vi "Event Handle Loop_Close Button.vi"(8 "error in (no error)":errorcluster, 10 "Label":string[](array[string]), 11 "QMenu Class in":refnum<class "QMenu Class.lvclass">) -> (0 "error out":errorcluster, 3 "QMenu Class out":refnum<class "QMenu Class.lvclass">)   [LabVIEW 2020, in "QTab.lvlib" / "QMenu Class.lvclass"]
uses:
  QMenu Class.lvclass
  QMenu Class.lvclass/QMenu Class.ctl
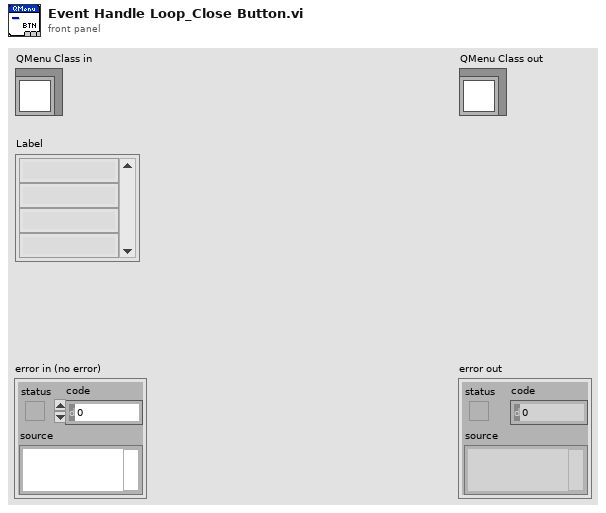
[diagram p1: front panel]
types:
  T1 = typedef "QTab.lvlib/QMenu Class.lvclass/Button Attribute.ctl" = cluster{"Label":string, "Button Text":string, "Closable":bool, "Draggable":bool}
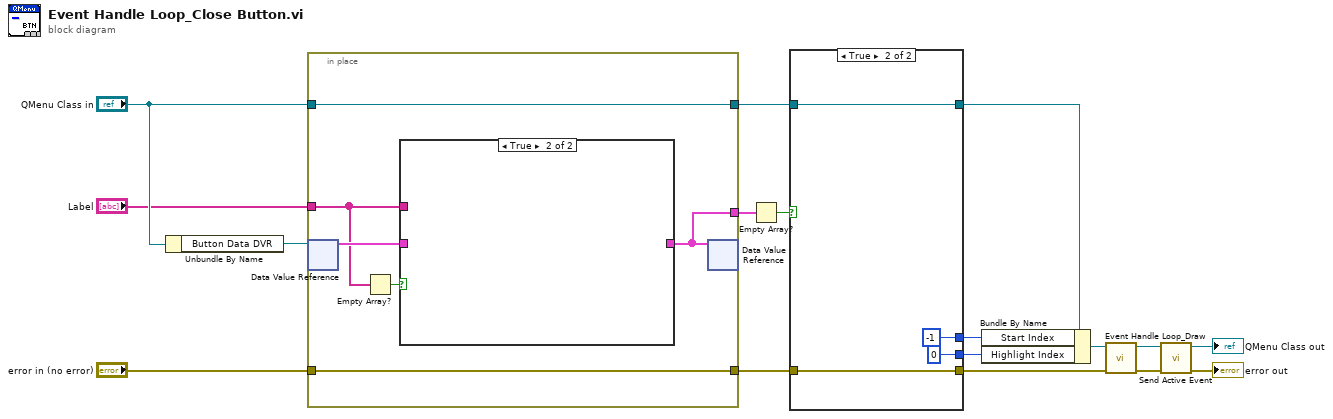
[diagram p0: block diagram]
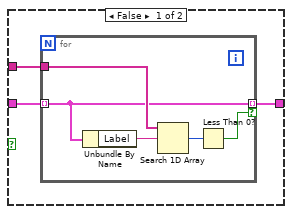
[diagram p3: hidden frame]
diagram:
  n1 = Unbundle By Name("QMenu Class in") -> ("Button Data DVR"=w17:refnum<data-value>)
  n2 = in-place {
    in-place-border: "QMenu Class in" -> [w23]
    in-place-border: [w23] -> w10
    in-place-border: "Label" -> [w18]
    in-place-border: "error in (no error)" -> [w22]
    in-place-border: [w22] -> w12
    in-place-border: [w19] -> w13
    n3 = in-place-dvr #1(w17) -> (w21:T1[])  [unwired: 1 out]
    n4 = Empty Array?(array=w18) -> (empty?=w20:bool)
    n5 = case shown="True" w20 {
      tunnel: w18 -> [w26 _]
      tunnel: [w25 _] -> w19
      tunnel: w21 -> [w24 _]
      frame False {
        n6 = for {
          tunnel: w24 -> [w29] mode=indexing
          tunnel: w26 -> [w30]
          tunnel: [w29] -> w25 mode=indexing if=w27
          n7 = Unbundle By Name(w29) -> ("Label"=w31:string)
          n8 = Search 1D Array(1D array=w30, element=w31) -> (index of element=w28:i32)  [unwired: 1 in]
          n9 = Less Than 0?(x=w28) -> (x < 0?=w27:bool)
        }
      }
      frame True {
      }
    }
    n10 = in-place-dvr #1(w19) -> ()  [unwired: 2 out]
  }
  n11 = Empty Array?(array=w13) -> (empty?=w11:bool)
  n12 = case shown="True" w11 {
    tunnel: w12 -> [w32 w36]
    tunnel: w10 -> [w33 w37]
    tunnel: [w33 w37] -> w9
    tunnel: [w32 w36] -> w6
    tunnel: [_ -1] -> w8
    tunnel: [_ 0] -> w7
    frame False {
    }
    frame True {
    }
  }
  n13 = Bundle By Name(cluster=w9, "Start Index"=w8, "Highlight Index"=w7) -> (w5:refnum<class "QMenu Class.lvclass">)
  n14 = call "Event Handle Loop_Draw.vi"("error in (no error)"=w6, "QMenu Class in"=w5) -> ("error out"=w3:errorcluster, "QMenu Class out"=w4:refnum<class "QMenu Class.lvclass">)  [unwired: 8 in]
  n15 = call "Send Active Event.vi"("error in (no error)"=w3, "QMenu Class in"=w4) -> ("error out"=→"error out":errorcluster, "QMenu Class out"=→"QMenu Class out":refnum<class "QMenu Class.lvclass">)  [unwired: 8 in]
